vi "Actor Core.vi"(8 "error in":errorcluster, 11 "[V] Tester Child in":refnum<class "[V] Tester Child.lvclass">) -> (0 "error out":errorcluster, 3 "Actor out":refnum<class "Actor.lvclass">)   [LabVIEW 2020, in "[V] Tester Child.lvlib" / "[V] Tester Child.lvclass"]
doc: "(<B>Filename</B>: Actor Framework.lvlib:Actor.lvclass:Actor Core.vi)\n\nReceives messages to the actor, reacts to them, and initiates any error handling that may shut the actor down.\n\nDescendant classes may override this VI to append parallel tasks for the actor to complete while it handles messages. Overrides use the Call Parent Class Method node."
uses:
  [V] Tester Child.lvclass
  C:/Program Files/National Instruments/LabVIEW 2020/vi.lib/ActorFramework/Actor/Actor.lvclass
  D:/2_GitHub/LabVIEW-MDI-Panel/[MDI] Child/[MDI] Child/[MDI] Child.lvclass
  <vilib>/ActorFramework/Actor/Actor.lvclass
  <vilib>/ActorFramework/Actor/Actor.lvclass/Actor.ctl
  <vilib>/ActorFramework/Message Enqueuer/Message Enqueuer.lvclass/Message Enqueuer.ctl
  [MDI] Child/[MDI] Child/[MDI] Child.lvclass/[MDI] Child.ctl
  <vilib>/numeric/Random Number (Range) DBL.vi
  [MDI] Child/[MDI] Child/Accessor/Read Child Name.vi
  <vilib>/ActorFramework/Message Enqueuer/Init from Existing Queue.vi
  <vilib>/ActorFramework/Message Enqueuer/Enqueue.vi
  <vilib>/ActorFramework/Stop Msg/Stop Msg.lvclass
  C:/Program Files/National Instruments/LabVIEW 2020/vi.lib/ActorFramework/Message/Message.lvclass
  <vilib>/ActorFramework/Message Priority Queue/Priority Enqueue.vi
  [MDI] Child/[MDI] Child/[MDI] Child.lvclass
  <vilib>/ActorFramework/Message Enqueuer/Message Enqueuer.lvclass
panel:
  out "chart":dbl(graph)
  # "Actor UI"
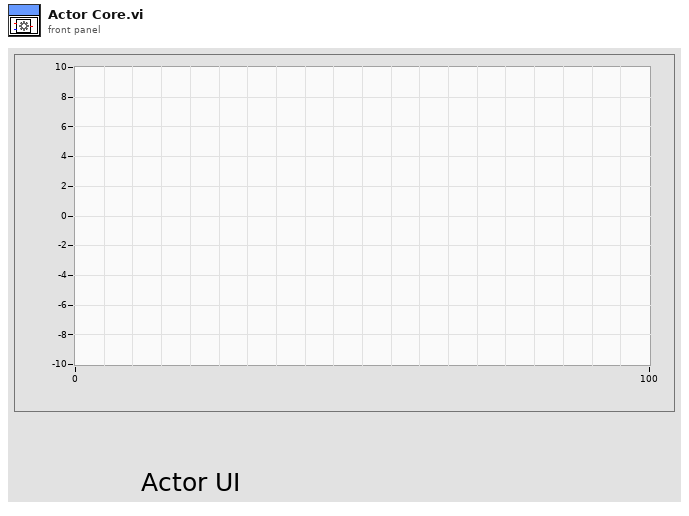
[diagram p1: front panel]
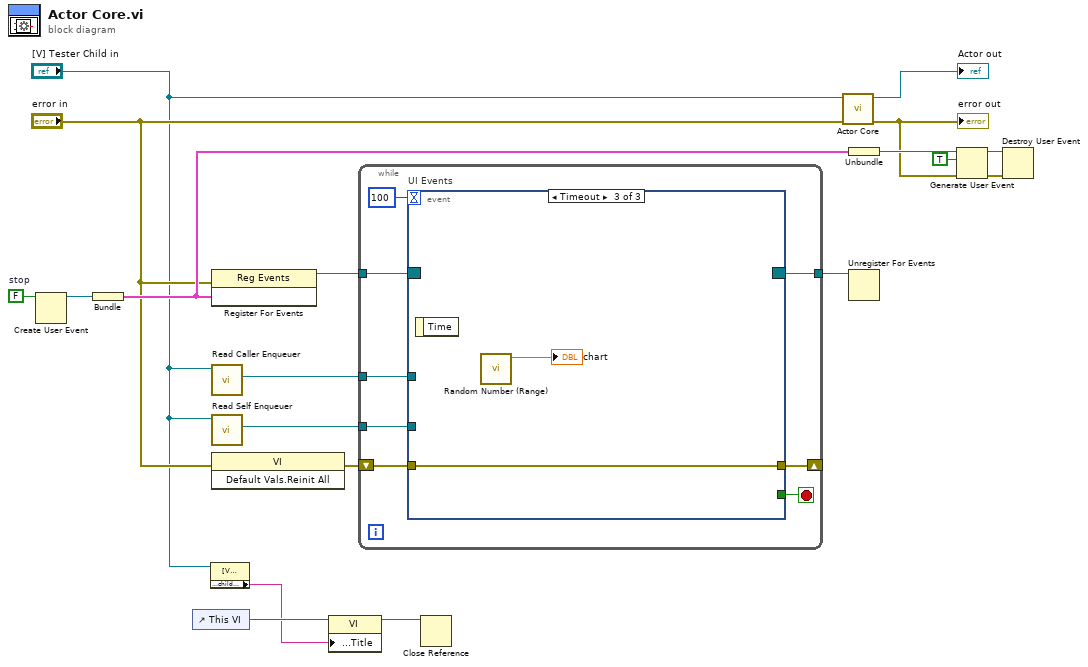
[diagram p0: block diagram]
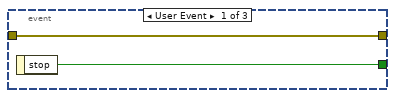
[diagram p2: hidden frame]
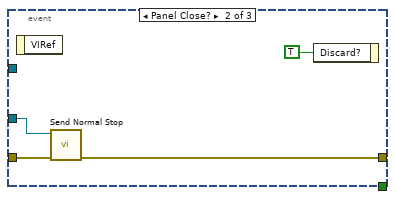
[diagram p3: hidden frame]
diagram:
  w9 = FALSE  # stop
  n1 = Create User Event(user event datatype=w9) -> (user event=w12:refnum<user-event>)  [unwired: 1 in, 1 out]
  n2 = Bundle("stop"=w12) -> (w13:cluster{"stop":refnum<user-event>})  [unwired: 1 in]
  n3 = control-ref of="This VI"() -> (w18:refnum<vi>)
  n4 = property class="[V] Tester Child.lvclass"(reference="[V] Tester Child in") -> ("Accessor:child name"=w17:string)  [unwired: 1 in, 2 out]
  n5 = register-events ("Main Register for Events")(error in="error in", w13) -> (reference out=w4:refnum<event-registration>)  [unwired: 1 in, 1 out]
  n6 = call <vilib>:"Read Caller Enqueuer.vi"("Actor"="[V] Tester Child in") -> ("Caller Enqueuer"=w7:refnum<class "Message Enqueuer.lvclass">)  [unwired: 10 in]
  n7 = call <vilib>:"Read Self Enqueuer.vi"("Actor"="[V] Tester Child in") -> ("Self Enqueuer"=w6:refnum<class "Message Enqueuer.lvclass">)  [unwired: 10 in]
  n8 = invoke class="VI" method="Default Vals.Reinit All"(error in="error in") -> (error out=w8:errorcluster)  [unwired: 2 in, 2 out]
  n9 = property class="VI"(reference=w18, "Front Panel.Title"=w17) -> (reference out=w16:refnum<vi>)  [unwired: 1 in, 1 out]
  n10 = while {
    tunnel: w4 -> [w27]
    tunnel: [w25] -> w5
    tunnel: w6 -> [w24]
    tunnel: w7 -> [w21]
    shift-right: [w22] -> _
    shift-left: w8 -> [w23]
    stop <- w26 stop-if-true
    n11 = event "UI Events" shown="[2] Timeout" {
      selector: w27 -> [_ _ _]
      dyn-events: [_ _ _] -> w25
      timeout: 100 -> [_ _ _]
      tunnel: [w28 _ _] -> w26
      tunnel: w24 -> [_ w32 _]
      tunnel: w23 -> [w29 w31 w34]
      tunnel: [w29 w30 w34] -> w22
      tunnel: w21 -> [_ _ _]
      event User Event {
        n12 = event-data() -> ("stop"=w28:bool)  [unwired: 1 in]
      }
      event Panel Close? {
        n13 = event-data() -> ()  [unwired: 1 in, 1 out]
        n14 = call <vilib>:"Send Normal Stop.vi"("error in (no error)"=w31, "Message Enqueuer"=w32) -> ("error out"=w30:errorcluster)  [unwired: 9 in]
        n15 = event-data("Discard?"=TRUE) -> ()  [unwired: 1 in, 1 out]
      }
      event Timeout {
        n16 = event-data() -> ()  [unwired: 1 in, 1 out]
        n17 = call-poly <vilib>:"Random Number (Range).vi"() -> ("number"=→"chart":dbl)  [unwired: 11 in]
      }
    }
  }
  n18 = Close Reference(reference=w16) -> ()  [unwired: 1 in, 1 out]
  n19 = call-parent "Actor Core.vi"("error in"="error in", "[MDI] Child in"="[V] Tester Child in") -> ("error out"=w2:errorcluster, "Actor out"=→"Actor out":refnum<class "Actor.lvclass">)  [unwired: 8 in]
  "error out" <- w2
  n20 = Unbundle(w13) -> ("stop"=w14:refnum<user-event>)
  n21 = Unregister For Events(event registration refnum=w5) -> ()  [unwired: 1 in, 1 out]
  n22 = Generate User Event(user event=w14, event data cluster=TRUE ("event data"), error in=w2) -> (user event out=w11:refnum<user-event>, error out=w15:errorcluster)  [unwired: 1 in]
  n23 = Destroy User Event(user event=w11, error in=w15) -> ()  [unwired: 1 out]
